vi "Digital Write Benchmark.vi"() -> ()   [LabVIEW 2011]
uses:
  Private/Type Defs/Peripherals/Digital/Digital Write Control.ctl
  Private/Type Defs/Interface.ctl
  Private/Device/Device.lvlib
  LVH-LINX.lvlib
  <vilib>/ptbypt/NI_PtbyPt.lvlib
panel:
  out "Loop Time (ms)":i32
  out "Loop Rate":dbl(graph)
  in  "Digital Values":T1[](array[typedef])=[{"Pin Number"=13, "Value"=TRUE}]
  in  "Stop Button":bool
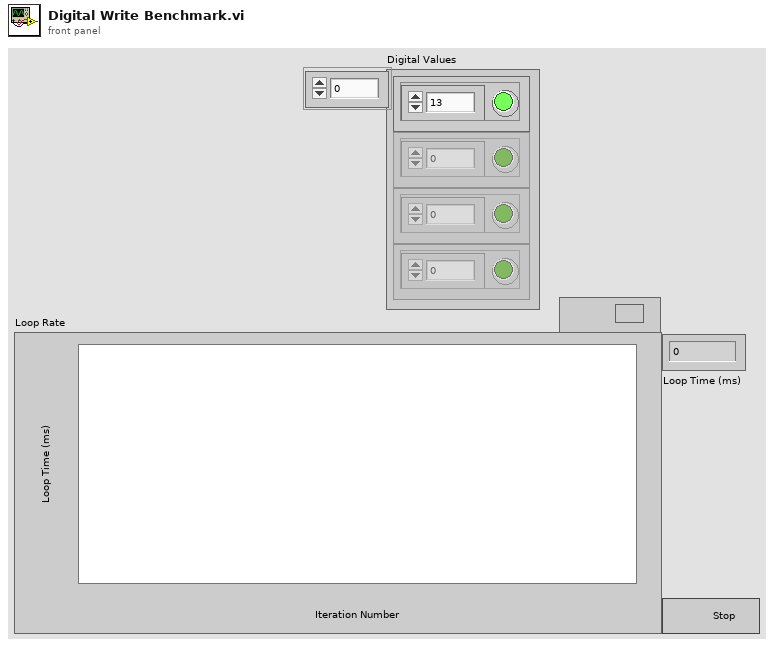
[diagram p1: front panel]
types:
  T1 = typedef "LVH-LINX.lvlib/Digital Write Control.ctl" = cluster{"Pin Number":u8, "Value":bool}
  T2 = typedef "LVH-LINX.lvlib/Interface.ctl" = enum16{"Serial", "TCP"}
  T3 = typedef "LVH-LINX.lvlib/Device.lvlib/LINX Device Config.ctl" = cluster{"Interface":T2, "COM Port":refnum<visa-resource-name>, "TCP Configuration":T4, "Device ID":u8, "Device Name":string, "Device Family":T5}
  T4 = typedef "LVH-LINX.lvlib/Device.lvlib/TCP Config.ctl" = cluster{"IP Address":string, "Port":dbl}
  T5 = typedef "LVH-LINX.lvlib/Device Family.ctl" = enum8{"National Instruments", "Digilent", "Arduino"}
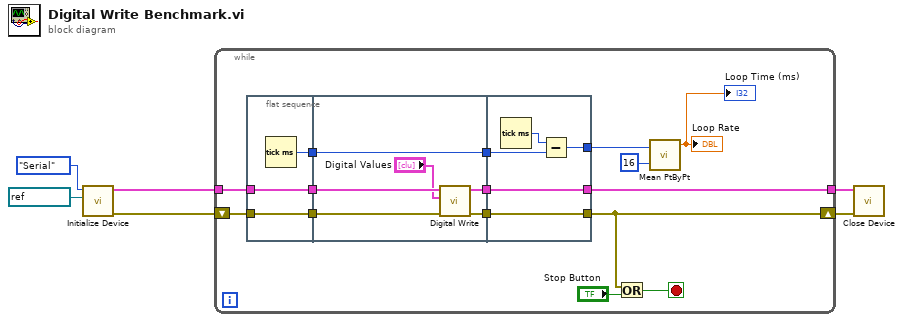
[diagram p0: block diagram]
diagram:
  n1 = call "Initialize Device.vi"("COM Port"=refnum<visa-resource-name> "COM5", "Interface"=Interface."Serial") -> ("Error Out"=w1:errorcluster, "LINX Device Config"=w2:T3)  [unwired: 8 in]
  n2 = while {
    tunnel: w2 -> [w20]
    tunnel: [w19] -> w3
    shift-right: [w17] -> w4
    shift-left: w1 -> [w21]
    stop <- w18 stop-if-true
    n3 = flat-sequence {
      tunnel: w20 -> [w23]
      tunnel: w21 -> [w24]
      tunnel: [w24] -> w15
      tunnel: [w23] -> w14
      tunnel: [w22] -> w11
      tunnel: w15 -> [w30]
      tunnel: w14 -> [w29]
      tunnel: [w28] -> w13
      tunnel: [w26] -> w12
      tunnel: w11 -> [w25]
      tunnel: [w25] -> w10
      tunnel: [w34] -> w17
      tunnel: [w35] -> w19
      tunnel: w13 -> [w35]
      tunnel: w12 -> [w34]
      tunnel: w10 -> [w32]
      tunnel: [w31] -> w9
      frame #0 {
        n4 = Tick Count (ms)() -> (millisecond timer value=w22:u32)
      }
      frame #1 {
        n5 = call "Digital Write.vi"("Error In"=w30, "Digital Values"="Digital Values", "LINX Device Config"=w29) -> ("Error Out"=w26:errorcluster, "LINX Device Config"=w28:T3)  [unwired: 7 in]
      }
      frame #2 {
        n6 = Tick Count (ms)() -> (millisecond timer value=w33:u32)
        n7 = Subtract(x=w33, y=w32) -> (x-y=w31:u32)
      }
    }
    n8 = Or(x=w17, y="Stop Button") -> (x .or. y?=w18:bool)
    n9 = call <vilib>:"Mean PtByPt.vi"("x"=w9, "sample length"=16) -> ("mean"=→"Loop Rate" →"Loop Time (ms)":dbl)  [unwired: 2 in, 1 out]
  }
  n10 = call "Close Device.vi"("Error In"=w4, "LINX Device Config"=w3) -> ()  [unwired: 8 in, 2 out]
